vi "Waveform_Extract from Start and End time with End point.vi"(8 "Error":errorcluster, 9 "End Time":dbl, 10 "Begin Time":dbl, 11 "Waveform":T1) -> (0 "Error Out":errorcluster, 1 "End Index Out":i32, 2 "Start Index Out":i32, 3 "Waveform Out":T1)   [LabVIEW 2016]
doc: "Retrieves a subset of a waveform at a specified time or index. You must manually select the polymorphic instance you want to use."
uses:
  Universal Controls/Waveform_Data.ctl
  Universal Controls/Read Write Button.ctl
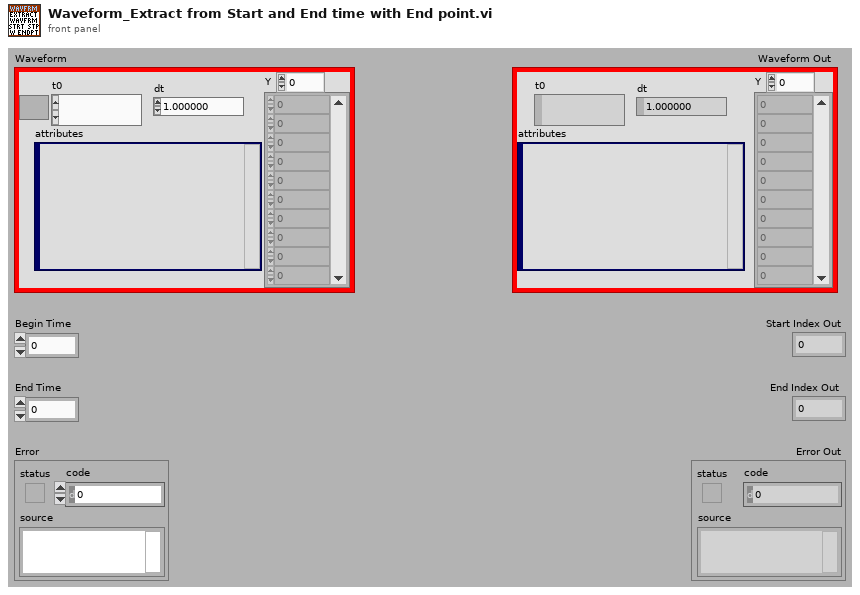
[diagram p1: front panel]
types:
  T1 = typedef "Waveform_Data.ctl" = waveform(dbl)
  T2 = typedef "Read Write Button.ctl" = bool
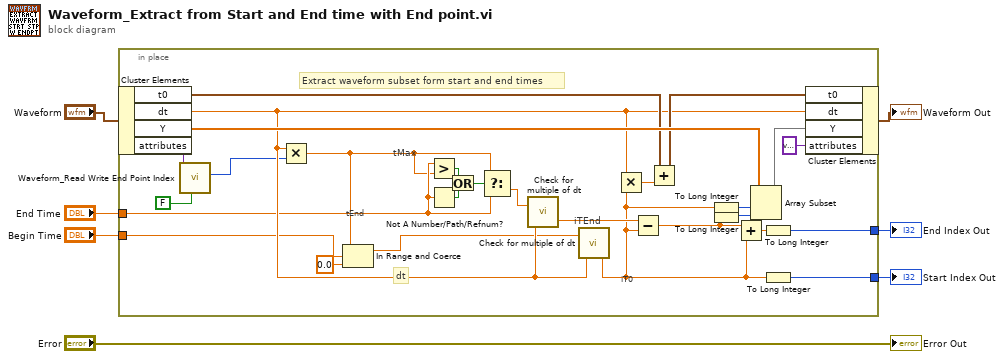
[diagram p0: block diagram]
diagram:
  n1 = in-place {
    in-place-border: "Begin Time" -> [w13]
    in-place-border: "End Time" -> [w18]
    in-place-border: [w30] -> w5
    in-place-border: [w29] -> w4
    # "Extract waveform subset form start and end times"
    # "dt"
    # "iTEnd"
    # "iT0"
    # "tEnd"
    # "tMax"
    n2 = in-place-cluster #1("Waveform") -> ("t0"=w21:timestamp, "dt"=w19:dbl, "Y"=w23:dbl[], "attributes"=w11:variant)
    n3 = call "Waveform_Read Write End Point Index.vi"("Read(f)\nWrite(t)"=T2 FALSE ("Read(f)\nWrite(t)"), "Waveform Atributes"=w11) -> ("End Point Out"=w9:i32)  [unwired: 7 in, 2 out]
    n4 = Multiply(x=w19, y=w9) -> (x*y=w15:dbl)
    n5 = In Range and Coerce(upper limit=w15, x=w13, lower limit=0.0) -> (coerced(x)=w12:dbl)  [unwired: 1 out]
    n6 = Greater?(x=w18, y=w15) -> (0:w34:bool)
    n7 = Not A Number/Path/Refnum?(number/path/refnum=w18) -> (NaN/Path/Refnum?=w33:bool)
    n8 = Or(x=w34, y=w33) -> (x .or. y?=w32:bool)
    n9 = Select(t=w15, s=w32, f=w18) -> (s? t:f=w16:dbl)
    n10 = call <vilib>:"Check for multiple of dt.vi"("dt"=w19, "time"=w16) -> ("iQuotient"=w31:dbl)  [unwired: 1 out]
    n11 = call <vilib>:"Check for multiple of dt.vi"("dt"=w19, "time"=w12) -> ("iQuotient"=w28:dbl)  [unwired: 1 out]
    n12 = Multiply(x=w19, y=w28) -> (x*y=w26:dbl)
    n13 = Subtract(x=w31, y=w28) -> (x-y=w17:dbl)
    n14 = Add(x=w21, y=w26) -> (x+y=w20:timestamp)
    n15 = To Long Integer(number=w28) -> (32bit integer=w24:i32)
    n16 = To Long Integer(number=w17) -> (32bit integer=w25:i32)
    n17 = Add(x=w17, y=w28) -> (x+y=w27:dbl)
    n18 = Array Subset(array=w23, index=w24, length=w25) -> (w22:dbl[])
    n19 = To Long Integer(number=w27) -> (32bit integer=w29:i32)
    n20 = To Long Integer(number=w28) -> (32bit integer=w30:i32)
    n21 = in-place-cluster #1("t0"=w20, "dt"=w19, "Y"=w22, "attributes"=variant) -> (→"Waveform Out":T1)
  }
  "Start Index Out" <- w5
  "End Index Out" <- w4
  "Error Out" <- "Error"
